vi "Global_KNRm.vi"() -> ()   [LabVIEW 2013]
panel:
  out "C_port":i8
  out "KLR":dbl
  out "CIRCLE":dbl
  in  "same pos":bool
  out "point":dbl
  out "1/2/3/4/5":i32
  out "X3":dbl
  out "deta 3":dbl[][](array[numeric])
  out "deta 2":dbl[][](array[numeric])
  out "deta 1":dbl[][](array[numeric])
  out "green":dbl
  out "X2":dbl
  out "X1":dbl
  out "xVcmd":dbl
  out "MoveDelay(ms)":dbl
  out "WWHL":i32
  out "dirN":i32[](array[numeric])
  out "dir_para":T1
  out "Move":T2
  out "revgain":i32
  out "V":dbl
  out "A":dbl
  out "J":dbl
  out "Jmax":i32
  out "Vmax":i32
  out "fs":i32
  out "Tcnt":dbl
  out "Ts":dbl
  out "Friction":dbl[](array[numeric])
  out "Kvi":dbl[](array[numeric])
  out "Kvp":dbl[](array[numeric])
  out "Kpp":dbl[](array[numeric])
  out "Kvff":dbl[](array[numeric])
  out "scKd":dbl
  out "scKi":dbl
  out "scKp":dbl
  out "PLS2DEG":dbl
  out "C2RNOF":dbl
  out "C2RFIX":dbl
  out "MM2DEG":dbl
  out "R_port":i8
  out "L_port":i8
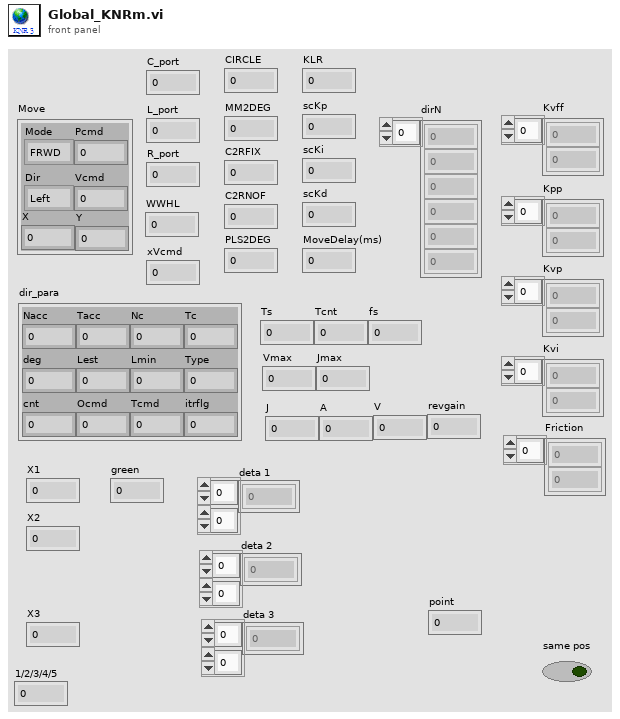
[diagram p1: front panel]
types:
  T1 = cluster{"Nacc":i32, "deg":dbl, "cnt":i32, "Tacc":dbl, "Lest":dbl, "Ocmd":dbl, "Nc":i32, "Lmin":dbl, "Tcmd":dbl, "Tc":dbl, "Type":i32, "itrflg":i32}
  T2 = cluster{"Pcmd":dbl, "Vcmd":dbl, "Mode":enum16{"FRWD", "TURFIX", "TURNOF", "CIRCULAR"}, "Dir":enum16{"Left", "Right"}, "Y":dbl, "X":dbl}
diagram:
